vi "Configure Pattern Mode.vi"(6 "Loop Offset (0)":i32, 7 "Number of Levels (2: 2 Levels)":i32(ring) items=["2 Levels", "3 Levels", "4 Levels"], 8 "error in (no error)":errorcluster, 9 "Bit Shape (0: NRZ Mode)":i32(ring) items=["NRZ Mode", "User Mode"], 10 "Enable Pattern Mode (F: Disable)":bool, 11 "VISA resource name":refnum<visa-resource-name>) -> (0 "error out":errorcluster, 3 "VISA resource name out":refnum<visa-resource-name>)   [LabVIEW 2009, in "Agilent 81150.lvlib"]
doc: "Configures general settings to pattern mode."
uses:
  Agilent 81150.lvlib
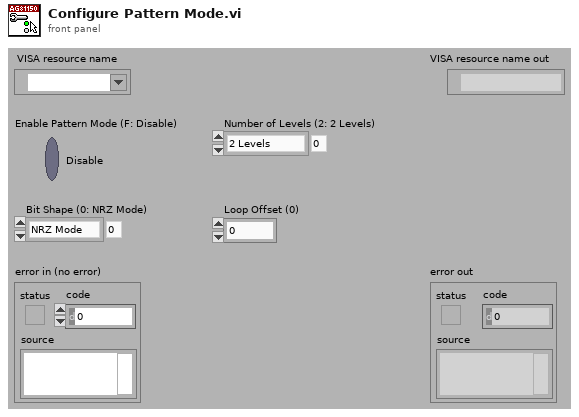
[diagram p1: front panel]
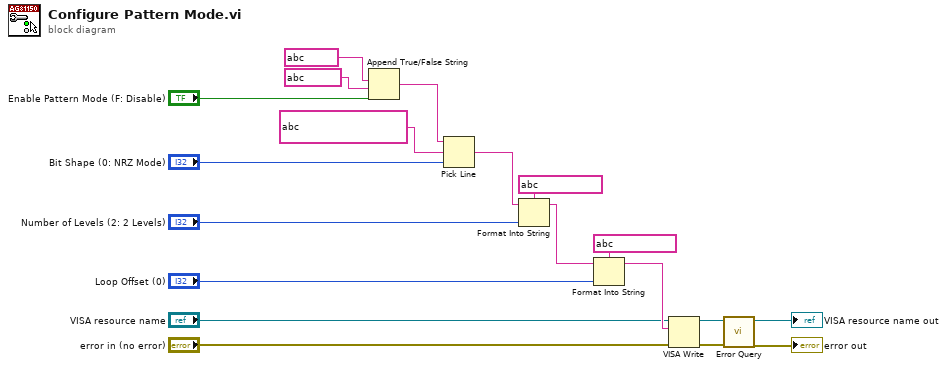
[diagram p0: block diagram]
diagram:
  n1 = Append True/False String(1:"Enable Pattern Mode (F: Disable)", 2:string ?, 3:string ?) -> (0:w14:string)  [unwired: 1 in]
  n2 = Pick Line(string ("")=w14, multi-line string=string ?, line index="Bit Shape (0: NRZ Mode)") -> (output string=w13:string)
  n3 = Format Into String(format string=string ?, initial string=w13, "Number of Levels (2: 2 Levels)") -> (resulting string=w10:string)  [unwired: 1 in, 1 out]
  n4 = Format Into String(format string=string ?, initial string=w10, "Loop Offset (0)") -> (resulting string=w7:string)  [unwired: 1 in, 1 out]
  n5 = VISA Write(VISA resource name="VISA resource name", write buffer=w7, error in (no error)="error in (no error)") -> (VISA resource name out=w4:refnum<visa-resource-name>, error out=w3:errorcluster)  [unwired: 1 out]
  n6 = call "Error Query.vi"("error in (no error)"=w3, "VISA resource name"=w4) -> ("error out"=→"error out":errorcluster, "VISA resource name out"=→"VISA resource name out":refnum<visa-resource-name>)  [unwired: 6 in, 2 out]
